vi "Kaelus PIM PIMHW Connection Daemon.vi"(8 "error in (no error)":errorcluster) -> (0 "error out":errorcluster)   [LabVIEW 2011]
uses:
  TypeDefs/Kaelus PIM PIMHW Connection CMDS.ctl
  PIM Configuration.ctl
  PIM Interface Language.ctl
panel:
  in  "PIM Configuration":T1={"host IP (localhost)"="localhost", "host Port"=3388, "Model"="", "Serial Number(s)"="", "Calibration Date"=3388.0, "Dual Port?"=FALSE, "DeviceNames"=[], "Parameters"={"TX1start"=0.0, "TX1stop"=0.0, "TX1pmax"=0.0, "TX2start"=0.0, "TX2stop"=0.0, "TX2pmax"=0.0, "RXstart"=0.0, "RXstop"=0.0}, "Interface"=enum."PIM Web Engine"} {"Calibration Date" format="%.2f"; "Parameters"."TX2pmax" format="%.1f"; "Parameters"."TX1pmax" format="%.1f"; "Parameters"."RXstop" format="%.1f"; "Parameters"."RXstart" format="%.1f"; "Parameters"."TX2stop" format="%.1f"; "Parameters"."TX2start" format="%.1f"; "Parameters"."TX1stop" format="%.1f"; "Parameters"."TX1start" format="%.1f"}
  in  "Timeout (30 mins)":dbl=30.0
  in  "PIMStatus":string
  out "ConnCmd":refnum<user-event>
  in  "Connection Command":T3
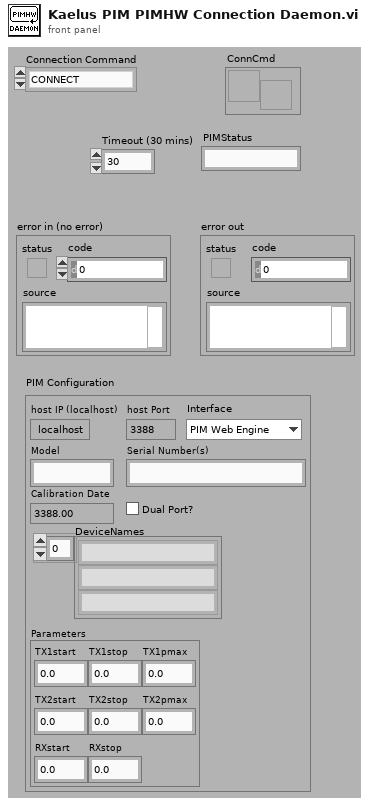
[diagram p1: front panel]
types:
  T1 = typedef "PIM Configuration.ctl" = cluster{"host IP (localhost)":string, "host Port":u16, "Model":string, "Serial Number(s)":string, "Calibration Date":dbl, "Dual Port?":bool, "DeviceNames":string[], "Parameters":cluster{"TX1start":dbl, "TX1stop":dbl, "TX1pmax":dbl, "TX2start":dbl, "TX2stop":dbl, "TX2pmax":dbl, "RXstart":dbl, "RXstop":dbl}, "Interface":T2}
  T2 = typedef "PIM Interface Language.ctl" = enum16{"PIM Web Engine", "PIM HW Engine"}
  T3 = typedef "Kaelus PIM PIMHW Connection CMDS.ctl" = enum16{"CONNECT", "DISCONNECT", "KEEP_ALIVE"}
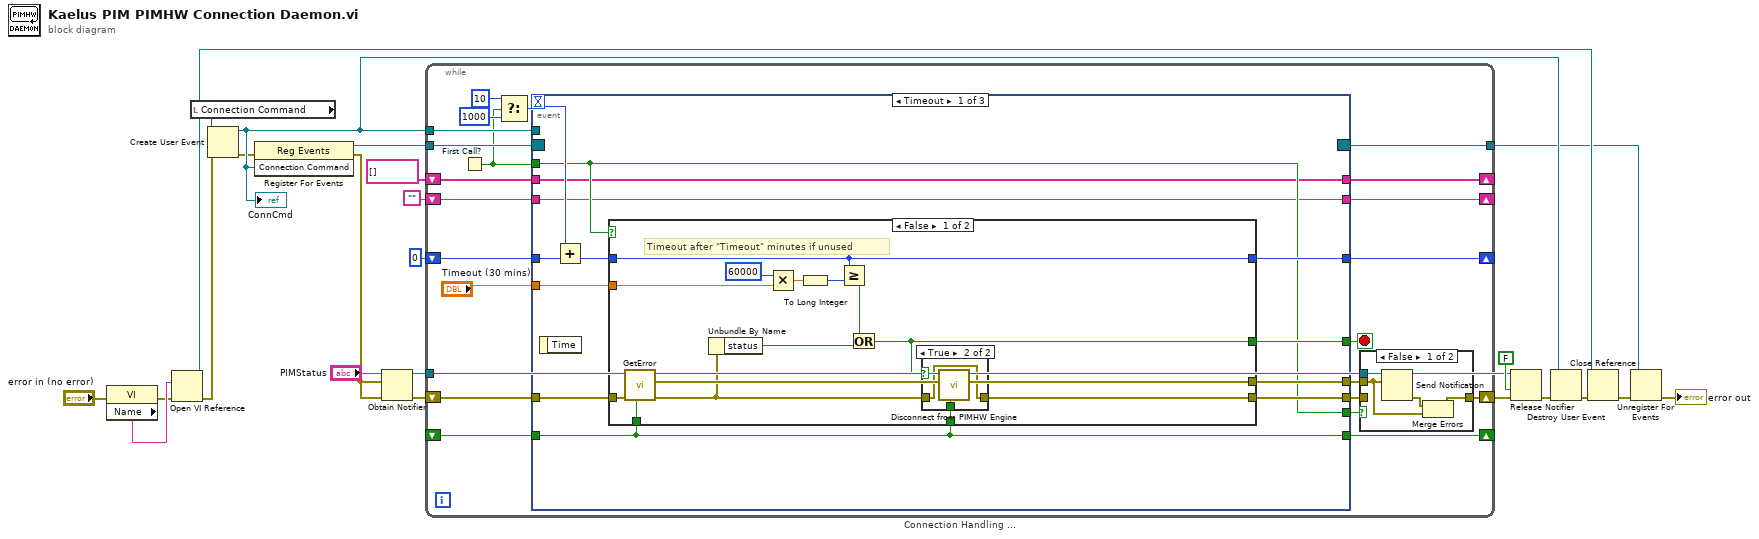
[diagram p0: block diagram]
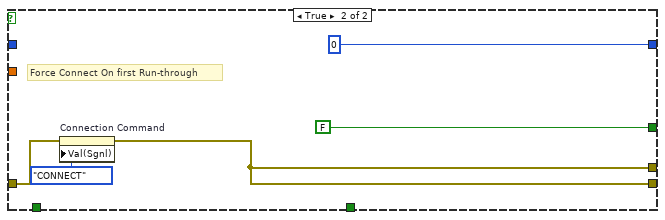
[diagram p4: hidden frame]
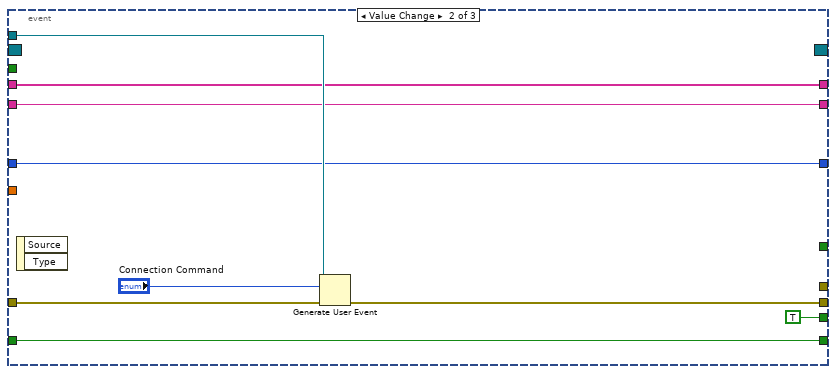
[diagram p5: hidden frame]
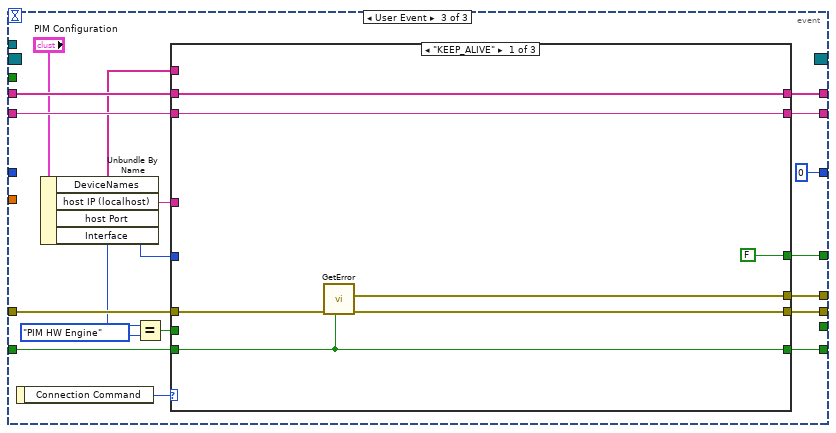
[diagram p6: hidden frame]
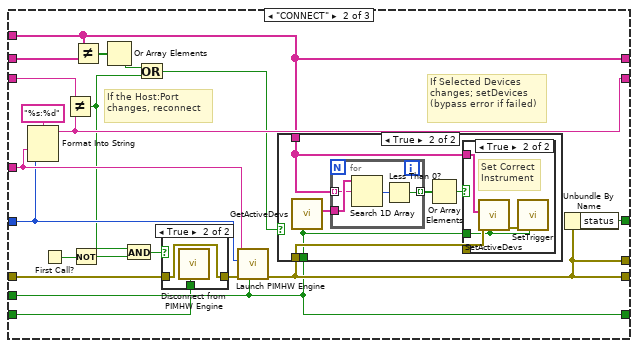
[diagram p7: hidden frame]
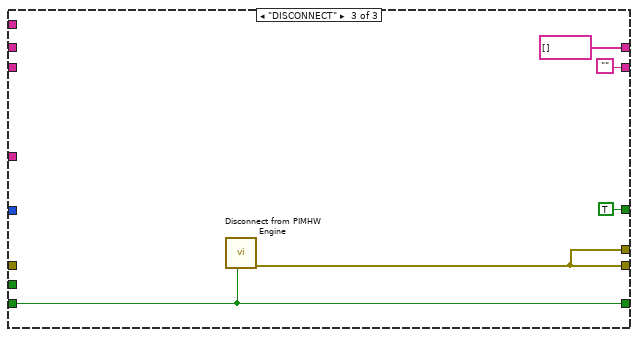
[diagram p11: hidden frame]
diagram:
  n1 = property class="VI"(error in="error in (no error)") -> (error out=w21:errorcluster, "Name"=w22:string)  [unwired: 1 in, 1 out]
  n2 = Open VI Reference(vi path=w22, error in (no error)=w21) -> (vi reference=w20:refnum<vi>, error out=w14:errorcluster)  [unwired: 4 out]
  n3 = local read "Connection Command"() -> (w18:T3)
  n4 = Create User Event(user event datatype=w18, error in=w14) -> (user event=w15:refnum<user-event>, error out=w13:errorcluster)
  "ConnCmd" <- w15
  n5 = register-events(error in=w13, w15) -> (reference out=w17:refnum<event-registration>, error out=w8:errorcluster)  [unwired: 1 in]
  n6 = Obtain Notifier(name (unnamed)="PIMStatus", notification data type=w8, error in (no error)=w8) -> (notifier out=w6:refnum<notifier>, error out=w7:errorcluster)  [unwired: 1 in, 1 out]
  n7 = while "Connection Handling ..." {
    shift-right: [w45] -> _
    shift-left: 0 -> [w46]
    tunnel: w17 -> [w43]
    shift-right: [w40] -> w11
    shift-left: w7 -> [w42]
    tunnel: w15 -> [w41]
    tunnel: w6 -> [w36]
    shift-right: [w30] -> _
    shift-left: "" -> [w31]
    shift-right: [w27] -> _
    shift-left: string[] [] ("Device Names 2") -> [w28]
    shift-right: [w26] -> _
    shift-left: _ -> [w25]
    tunnel: [w24] -> w1
    stop <- w44 stop-if-true
    n8 = First Call?() -> (First Call?: T/F=w33:bool)
    n9 = Select(t=10, s=w33, f=1000) -> (s? t:f=w32:i32)
    n10 = event shown="[0] Timeout" {
      selector: w43 -> [_ _ _]
      dyn-events: [_ _ _] -> w24
      timeout: w32 -> [w63 _ _]
      tunnel: w46 -> [w64 w91 _]
      tunnel: [w60 w91 0] -> w45
      tunnel: [w61 _ w111] -> w44
      tunnel: w42 -> [w59 w93 w113]
      tunnel: [w58 w92 w109] -> w39
      tunnel: w41 -> [_ w95 _]
      tunnel: w33 -> [w56 _ _]
      tunnel: [w57 _ w110] -> w38
      tunnel: [w56 TRUE ("First Call?: T/F") _] -> w37
      tunnel: w31 -> [w55 w89 w108]
      tunnel: [w55 w89 w107] -> w30
      tunnel: "Timeout (30 mins)" -> [w54 _ _]
      tunnel: w28 -> [w53 w88 w106]
      tunnel: [w53 w88 w105] -> w27
      tunnel: [w52 w87 w97] -> w26
      tunnel: w25 -> [w52 w87 w96]
      event Timeout {
        n11 = event-data() -> ()  [unwired: 2 out]
        n12 = Add(x=w63, y=w64) -> (x+y=w62:i32)
        n13 = case shown="False" w56 {
          tunnel: w62 -> [w77 _]
          tunnel: [w67 FALSE] -> w61
          tunnel: [w77 0] -> w60
          tunnel: w59 -> [w75 w84]
          tunnel: [w68 w82] -> w58
          tunnel: [w70 w82] -> w57
          tunnel: w54 -> [w73 _]
          tunnel: w52 -> [w71 _]
          tunnel: w52 -> [w66 _]
          frame False {
            # "Timeout after \"Timeout\" minutes if unused"
            n14 = call "GetError.vi"("Legacy (f)?"=w71, "error in (no error)"=w75) -> ("error out"=w69:errorcluster, "HW Error"=w70:errorcluster)  [unwired: 8 out]
            n15 = Unbundle By Name(w69) -> ("status"=w76:bool)
            n16 = Multiply(x=60000, y=w73) -> (x*y=w72:dbl)
            n17 = To Long Integer(number=w72) -> (32bit integer=w65:i32)
            n18 = Greater Or Equal?(x=w77, y=w65) -> (x >= y?=w78:bool)
            n19 = Or(x=w78, y=w76) -> (x .or. y?=w67:bool)
            n20 = case shown="True" w67 {
              tunnel: w69 -> [w79 w81]
              tunnel: [w79 w81] -> w68
              tunnel: w66 -> [_ w80]
              frame False {
              }
              frame True {
                n21 = call "Disconnect from PIMHW Engine.vi"("Legacy (f)?"=w80) -> ()  [unwired: 10 in, 1 out]
              }
            }
          }
          frame True {
            # "Force Connect On first Run-through"
            n22 = property on="Connection Command" class="Enum (strict)"(error in=w84, "Val(Sgnl)"=Kaelus_PIM_PIMHW_Connection_CMDS."CONNECT" ("Value (Signaling)")) -> (error out=w82:errorcluster)  [unwired: 1 in, 1 out]
          }
        }
      }
      event Value Change {
        n23 = event-data() -> ()  [unwired: 3 out]
        n24 = Generate User Event(user event=w95, event data cluster="Connection Command", error in=w93) -> (error out=w92:errorcluster)  [unwired: 1 out]
      }
      event User Event {
        n25 = event-data() -> ("Connection Command"=w114:T3)  [unwired: 1 out]
        n26 = Unbundle By Name("PIM Configuration") -> ("DeviceNames"=w104:string[], "host IP (localhost)"=w103:string, "host Port"=w102:u16, "Interface"=w99:T2)
        n27 = Equal?(x=w99, y=PIM_Interface_Language."PIM HW Engine" ("Interface")) -> (x = y?=w98:bool)
        n28 = case shown="\"KEEP_ALIVE\"" w114 {
          tunnel: w113 -> [w120 w136 _]
          tunnel: [w119 w134 w162] -> w109
          tunnel: [FALSE ("status") w141 TRUE ("status")] -> w111
          tunnel: [w118 w134 w162] -> w110
          tunnel: w103 -> [_ w140 _]
          tunnel: w108 -> [w117 w137 _]
          tunnel: [w117 w138 ""] -> w107
          tunnel: w104 -> [_ w129 _]
          tunnel: w106 -> [w116 w133 _]
          tunnel: [w116 w129 string[] [] ("Device Names 2")] -> w105
          tunnel: w102 -> [_ w128 _]
          tunnel: w98 -> [_ w123 _]
          tunnel: [w115 w123 w159] -> w97
          tunnel: w96 -> [w115 w122 w159]
          frame "KEEP_ALIVE" {
            n29 = call "GetError.vi"("Legacy (f)?"=w115, "error in (no error)"=w120) -> ("error out"=w119:errorcluster, "HW Error"=w118:errorcluster)  [unwired: 8 out]
          }
          frame "CONNECT" {
            # "If Selected Devices changes; setDevices\n(bypass error if failed)"
            # "If the Host:Port changes, reconnect"
            n30 = Format Into String(format string="%s:%d", w140, w128) -> (resulting string=w138:string)  [unwired: 2 in, 1 out]
            n31 = First Call?() -> (First Call?: T/F=w125:bool)
            n32 = Not Equal?(x=w137, y=w138) -> (x != y?=w126:bool)
            n33 = Not(x=w125) -> (.not. x?=w124:bool)
            n34 = Not Equal?(x=w129, y=w133) -> (x != y?=w132:bool[])
            n35 = Or Array Elements(Boolean array=w132) -> (logical OR=w131:bool)
            n36 = And(x=w126, y=w124) -> (x .and. y?=w127:bool)
            n37 = Or(x=w131, y=w126) -> (x .or. y?=w130:bool)
            n38 = case shown="True" w127 {
              tunnel: w136 -> [w156 w158]
              tunnel: [w156 w158] -> w135
              tunnel: w122 -> [_ w157]
              frame False {
              }
              frame True {
                n39 = call "Disconnect from PIMHW Engine.vi"("Legacy (f)?"=w157) -> ()  [unwired: 10 in, 1 out]
              }
            }
            n40 = call "Launch PIMHW Engine.vi"("Legacy (f)?"=w123, "error in (no error)"=w135, "port (80)"=w128, "host (localhost)"=w140) -> ("error out"=w134:errorcluster)  [unwired: 3 in, 4 out]
            n41 = case shown="True" w130 {
              tunnel: w134 -> [_ w147]
              tunnel: w129 -> [_ w142]
              tunnel: w123 -> [_ w146]
              frame False {
              }
              frame True {
                n42 = call "GetActiveDevs.vi"("Legacy (f)?"=w146) -> ("Active Device Names"=w145:string[])  [unwired: 9 in, 1 out]
                n43 = for {
                  tunnel: w142 -> [w154] mode=indexing
                  tunnel: w145 -> [w155]
                  tunnel: [w152] -> w144 mode=indexing
                  n44 = Search 1D Array(1D array=w155, element=w154) -> (index of element=w153:i32)  [unwired: 1 in]
                  n45 = Less Than 0?(x=w153) -> (x < 0?=w152:bool)
                }
                n46 = Or Array Elements(Boolean array=w144) -> (logical OR=w143:bool)
                n47 = case shown="True" w143 {
                  tunnel: w147 -> [_ w151]
                  tunnel: w146 -> [_ w149]
                  tunnel: w142 -> [_ w148]
                  frame False {
                  }
                  frame True {
                    # "Set Correct\nInstrument"
                    n48 = call "SetActiveDevs.vi"("Legacy (f)?"=w149, "error in (no error)"=w151, "Device DAQmx Names"=w148) -> ("error out"=w150:errorcluster)  [unwired: 8 in]
                    n49 = call "SetTrigger.vi"("Legacy (f)?"=w149, "error in (no error)"=w150) -> ()  [unwired: 9 in, 1 out]
                  }
                }
              }
            }
            n50 = Unbundle By Name(w134) -> ("status"=w141:bool)
          }
          frame "DISCONNECT" {
            n51 = call "Disconnect from PIMHW Engine.vi"("Legacy (f)?"=w159) -> ("error out"=w162:errorcluster)  [unwired: 10 in]
          }
        }
      }
    }
    n52 = case shown="False" w37 {
      tunnel: [w47 w51] -> w40
      tunnel: w39 -> [_ w51]
      tunnel: w38 -> [w48 _]
      tunnel: w36 -> [w50 _]
      frame False {
        n53 = Send Notification(notification=w48, notifier=w50) -> (error out=w49:errorcluster)  [unwired: 1 in, 1 out]
        n54 = Merge Errors(w49, w48) -> (w47:errorcluster)
      }
      frame True {
      }
    }
  }
  n55 = Release Notifier(notifier=w6, force destroy? (F)=FALSE, error in (no error)=w11) -> (error out=w12:errorcluster)  [unwired: 2 out]
  n56 = Destroy User Event(user event=w15, error in=w12) -> (error out=w16:errorcluster)
  n57 = Close Reference(reference=w20, error in (no error)=w16) -> (error out=w3:errorcluster)
  n58 = Unregister For Events(event registration refnum=w1, error in=w3) -> (error out=→"error out":errorcluster)
